vi "ComunicacionSerial.vi"() -> ()   [LabVIEW 2020]
uses:
  <vilib>/Instr/_visa.llb/VISA Configure Serial Port (Instr).vi
  <vilib>/ErrorRing/Error Ring.xnode
panel:
  out "Boolean":bool
  out "RX":string
  in  "TX":string
  in  "Config Serial":T1={"Puerto Serial"="", "Baudios"=9600, "Data Bis"=8, "Paridad"=enum."None", "Bits Stop"=10, "Control"=0} {"Control" items=["None", "XON/XOFF", "RTS/CTS", "XON/XOFF & RTS/CTS", "DTR/DSR", "XON/XOFF & DTR/DSR"]; "Bits Stop" items=["1.0"=10, "1.5"=15, "2.0"=20]; "Data Bis" min=5 max=8 step=1}
  in  "?":bool
  # "Comunicación Serial"
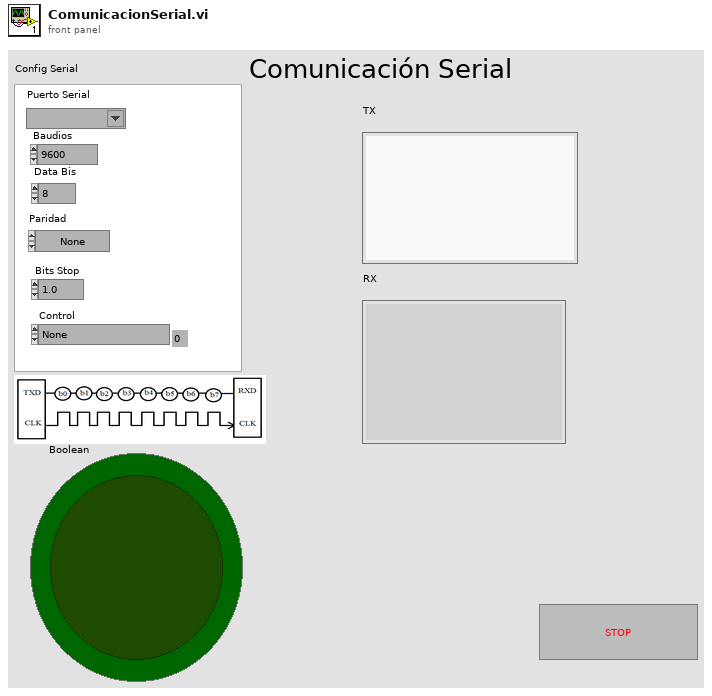
[diagram p1: front panel]
types:
  T1 = cluster{"Puerto Serial":refnum<visa-resource-name>, "Baudios":u32, "Data Bis":u16, "Paridad":enum16{"None", "Odd", "Even", "Mark", "Space"}, "Bits Stop":u16, "Control":u16}
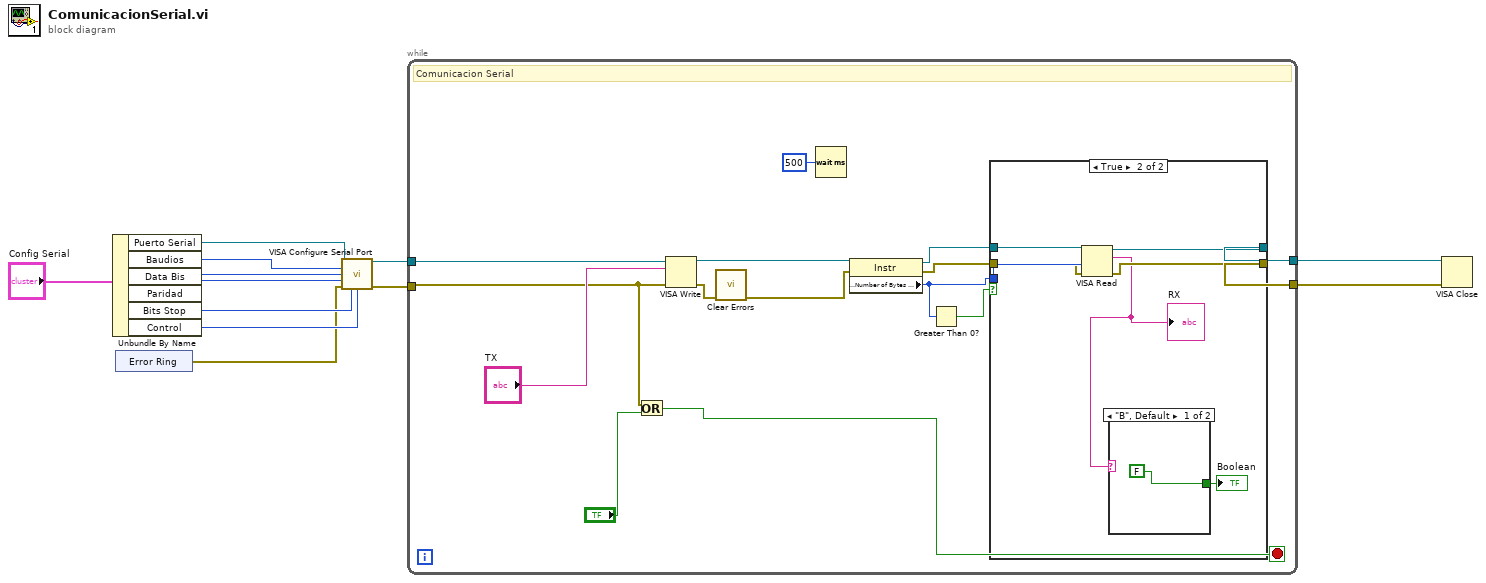
[diagram p0: block diagram]
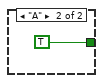
[diagram p3: hidden frame]
diagram:
  n1 = Unbundle By Name("Config Serial") -> ("Puerto Serial"=w11:refnum<visa-resource-name>, "Baudios"=w10:u32, "Data Bis"=w9:u16, "Paridad"=w8:enum16{"None", "Odd", "Even", "Mark", "Space"}, "Bits Stop"=w7:u16, "Control"=w6:u16)
  n2 = xnode "Error Ring"() -> ("error out"=w5:errorcluster)
  n3 = call-poly "VISA Configure Serial Port"("VISA resource name"=w11, "baud rate (9600)"=w10, "data bits (8)"=w9, "parity (0:none)"=w8, "error in (no error)"=w5, "stop bits (10: 1 bit)"=w7, "flow control (0:none)"=w6) -> ("VISA resource name out"=w4:refnum<visa-resource-name>, "error out"=w3:errorcluster)  [unwired: 7 in]
  n4 = while {
    tunnel: w4 -> [w27]
    tunnel: w3 -> [w23]
    tunnel: [w15] -> w2
    tunnel: [w14] -> w1
    stop <- w21 stop-if-true
    # "Comunicacion Serial"
    n5 = Or(x=w23, y="?") -> (x .or. y?=w21:bool)
    n6 = VISA Write(VISA resource name=w27, write buffer="TX", error in (no error)=w23) -> (VISA resource name out=w20:refnum<visa-resource-name>, error out=w24:errorcluster)  [unwired: 1 out]
    n7 = call <vilib>:"Clear Errors.vi"("error in (no error)"=w24) -> ("error out"=w19:errorcluster)  [unwired: 5 in, 1 out]
    n8 = Wait (ms)(milliseconds to wait=u32 500) -> ()  [unwired: 1 out]
    n9 = property class="Instr"(reference=w20, error in=w19) -> (reference out=w17:refnum<visa-resource-name>, error out=w16:errorcluster, "Serial Settings:Number of Bytes at Serial Port"=w13:u32)
    n10 = Greater Than 0?(x=w13) -> (x > 0?=w18:bool)
    n11 = case shown="True" w18 {
      tunnel: [w29 w32] -> w15
      tunnel: w17 -> [w29 w36]
      tunnel: w16 -> [w28 w34]
      tunnel: [w28 w33] -> w14
      tunnel: w13 -> [_ w35]
      frame False {
      }
      frame True {
        n12 = VISA Read(VISA resource name=w36, byte count=w35, error in (no error)=w34) -> (VISA resource name out=w32:refnum<visa-resource-name>, read buffer=w31:string, error out=w33:errorcluster)  [unwired: 1 out]
        "RX" <- w31
        n13 = case shown="\"B\", Default" w31 {
          tunnel: [FALSE TRUE] -> w30
          frame "B", Default {
          }
          frame "A" {
          }
        }
        "Boolean" <- w30
      }
    }
  }
  n14 = VISA Close(VISA resource name=w2, error in (no error)=w1) -> ()  [unwired: 1 out]
